vi "Parse Cors Rule.vi"(11 "String":string) -> (3 "Cors rule":T1)   [LabVIEW 2015, in "NI_Azure_Queue.lvlib"]
uses:
  NI_Azure_Queue.lvlib
  Cors Rule.ctl
  XML Parsing/NI_Azure_XML Parsing.lvlib
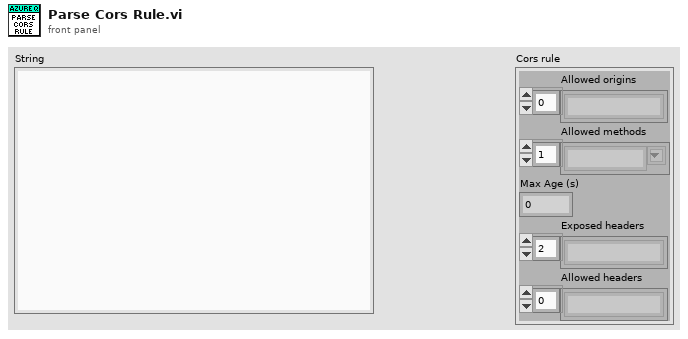
[diagram p1: front panel]
types:
  T1 = typedef "NI_Azure_Queue.lvlib/Cors Rule.ctl" = cluster{"Allowed origins":string[], "Allowed methods":string[], "Max Age (s)":u32, "Exposed headers":string[], "Allowed headers":string[]}
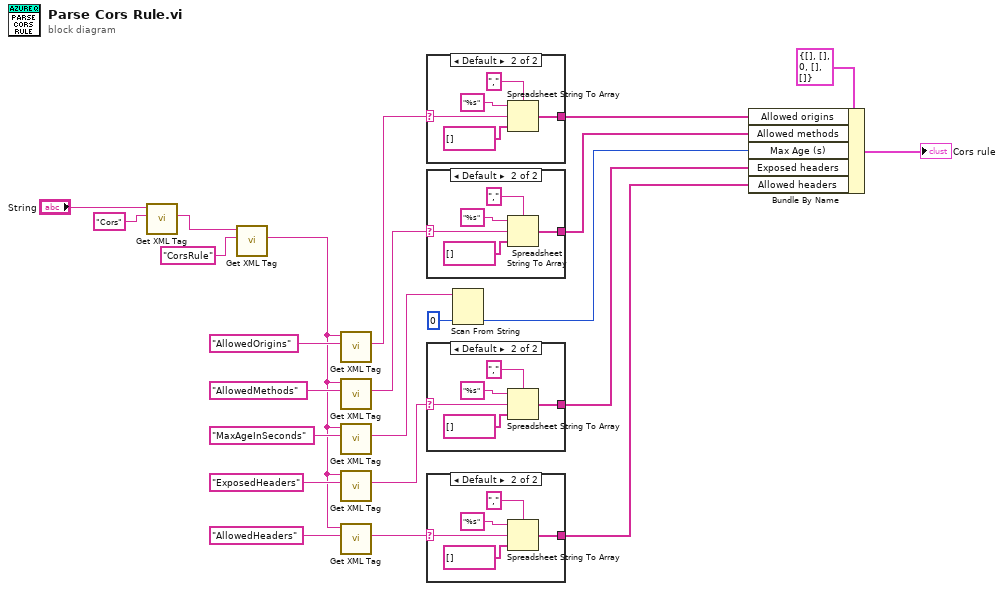
[diagram p0: block diagram]
diagram:
  n1 = call "Get XML Tag.vi"("Tag name"="Cors", "XML String in"="String") -> ("Tag value"=w14:string)  [unwired: 5 in, 4 out]
  n2 = call "Get XML Tag.vi"("Tag name"="CorsRule", "XML String in"=w14) -> ("Tag value"=w13:string)  [unwired: 5 in, 4 out]
  n3 = call "Get XML Tag.vi"("Tag name"="AllowedOrigins", "XML String in"=w13) -> ("Tag value"=w8:string)  [unwired: 5 in, 4 out]
  n4 = call "Get XML Tag.vi"("Tag name"="AllowedMethods", "XML String in"=w13) -> ("Tag value"=w6:string)  [unwired: 5 in, 4 out]
  n5 = call "Get XML Tag.vi"("Tag name"="MaxAgeInSeconds", "XML String in"=w13) -> ("Tag value"=w17:string)  [unwired: 5 in, 4 out]
  n6 = call "Get XML Tag.vi"("Tag name"="ExposedHeaders", "XML String in"=w13) -> ("Tag value"=w4:string)  [unwired: 5 in, 4 out]
  n7 = call "Get XML Tag.vi"("Tag name"="AllowedHeaders", "XML String in"=w13) -> ("Tag value"=w2:string)  [unwired: 5 in, 4 out]
  n8 = case shown="Default" w8 {
    selector: w8 -> [_ w28]
    tunnel: [_ w24] -> w7
    frame "" {
    }
    frame Default {
      n9 = Spreadsheet String To Array(delimiter (Tab)=",", format string="%s", spreadsheet string=w28, array type (2D Dbl)=string[] []) -> (array=w24:string[])
    }
  }
  n10 = case shown="Default" w6 {
    selector: w6 -> [_ w33]
    tunnel: [_ w29] -> w5
    frame "" {
    }
    frame Default {
      n11 = Spreadsheet String To Array(delimiter (Tab)=",", format string="%s", spreadsheet string=w33, array type (2D Dbl)=string[] []) -> (array=w29:string[])
    }
  }
  n12 = case shown="Default" w4 {
    selector: w4 -> [_ w38]
    tunnel: [_ w34] -> w3
    frame "" {
    }
    frame Default {
      n13 = Spreadsheet String To Array(delimiter (Tab)=",", format string="%s", spreadsheet string=w38, array type (2D Dbl)=string[] []) -> (array=w34:string[])
    }
  }
  n14 = case shown="Default" w2 {
    selector: w2 -> [_ w43]
    tunnel: [_ w39] -> w1
    frame "" {
    }
    frame Default {
      n15 = Spreadsheet String To Array(delimiter (Tab)=",", format string="%s", spreadsheet string=w43, array type (2D Dbl)=string[] []) -> (array=w39:string[])
    }
  }
  n16 = Scan From String(input string=w17, default 1=u32 0 ("Max Age (s)")) -> (output 1=w9:u32)  [unwired: 3 in, 3 out]
  n17 = Bundle By Name(cluster=T1 {"Allowed origins"=[], "Allowed methods"=[], "Max Age (s)"=0, "Exposed headers"=[], "Allowed headers"=[]} ("Cors rule"), "Allowed origins"=w7, "Allowed methods"=w5, "Max Age (s)"=w9, "Exposed headers"=w3, "Allowed headers"=w1) -> (→"Cors rule":T1)
